vi "Begin.vi"() -> (0 "error out":errorcluster)   [LabVIEW 2012]
doc: "Called before other user functions, this VI is expected to open initial I/O refnums, load in file data, and do all program initialization. Notice that the <B>error out</B> terminal is simply used for data flow. Wiring it to other structures or subVIs ensures that this VI runs first."
uses:
  <vilib>/Rock Robotics/WPI/DriverStation/WPI_DriverStationRobotMode2.ctl
  <vilib>/Rock Robotics/WPI/Joystick/WPI_JoystickDeviceEnum.ctl
  <vilib>/Rock Robotics/WPI/Solenoid/WPI_SolenoidChannel.ctl
  <vilib>/Rock Robotics/SystemInterfaces/DIO/FPGA_DIOChannel.ctl
  <vilib>/Rock Robotics/WPI/Encoder/WPI_EncoderType.ctl
  <vilib>/Rock Robotics/SystemInterfaces/DIO/FPGA_DIOPWMChannel.ctl
  <vilib>/Rock Robotics/SystemInterfaces/DIO/FPGA_DIORelayChannel.ctl
  <vilib>/Rock Robotics/SystemInterfaces/AI/FPGA_AIGyroChannel.ctl
  Robot Global Data.vi
  <vilib>/Rock Robotics/WPI/Solenoid/WPI_SolenoidOpenSingle.vi
  <vilib>/Rock Robotics/WPI/Solenoid/Deprecated/WPI_SolenoidSetBool.vi
  <vilib>/Rock Robotics/WPI/Counter/WPI_CounterDigitalInputToDigitalSource.vi
  <vilib>/Rock Robotics/WPI/MotorControl/WPI_MotorControlOpen Jaguar.vi
  <vilib>/Rock Robotics/WPI/RobotDrive/WPI_RobotDriveOpen4MotorWithTalon.vi
  <vilib>/Rock Robotics/WPI/Compressor/WPI_CompressorGetSetRefNum.vi
  <vilib>/Rock Robotics/WPI/MotorControl/WPI_MotorControlOpen Talon.vi
  <vilib>/Rock Robotics/WPI/MotorControl/WPI_MotorControlOpen Victor.vi
  <vilib>/Rock Robotics/WPI/RobotDrive/WPI_RobotDriveOpen4MotorWithExistingMotors.vi
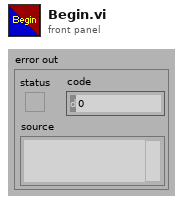
[diagram p1: front panel]
types:
  T1 = typedef "FPGA_DIOPWMChannel.ctl" = enum8{"PWM 1", "PWM 2", "PWM 3", "PWM 4", "PWM 5", "PWM 6", "PWM 7", "PWM 8", "PWM 9", "PWM 10", "Invalid"}
  T2 = typedef "FPGA_DIOChannel.ctl" = enum8{"DIO 1", "DIO 2", "DIO 3", "DIO 4", "DIO 5", "DIO 6", "DIO 7", "DIO 8", "DIO 9", "DIO 10", "DIO 11", "DIO 12", "DIO 13", "DIO 14", "Invalid"}
  T3 = typedef "WPI_SolenoidChannel.ctl" = enum8{"Solenoid 1", "Solenoid 2", "Solenoid 3", "Solenoid 4", "Solenoid 5", "Solenoid 6", "Solenoid 7", "Solenoid 8", "Invalid"}
  T4 = typedef "FPGA_AIGyroChannel.ctl" = enum8{"AI 1", "AI 2", "Invalid"}
  T5 = typedef "WPI_EncoderType.ctl" = enum16{"1x", "2x", "4x"}
  T6 = typedef "FPGA_DIORelayChannel.ctl" = enum8{"Relay 1", "Relay 2", "Relay 3", "Relay 4", "Relay 5", "Relay 6", "Relay 7", "Relay 8", "Invalid"}
  T7 = typedef "WPI_JoystickDeviceEnum.ctl" = enum16{"USB 1", "USB 2", "USB 3", "USB 4", "Kinect 1", "Kinect 2"}
  T8 = typedef "WPI_DriverStationRobotMode2.ctl" = enum16{"Autonomous Disabled", "Autonomous Enabled", "Teleop Disabled", "Teleop Enabled", "Timeout", "Finish", "Test Disabled", "Test Enabled"}
  T9 = typedef "WPI_RobotDriveDevRef.ctl" = cluster{"DevStatus":errorcluster, "Motors[]":T10[], "Square Inputs":bool, "Max Output":dbl, "Isochronous":bool}
  T10 = typedef "WPI_MotorControlDeviceRef.ctl" = cluster{"DeviceStatus":errorcluster, "Type":enum16{"PWM", "CAN"}, "PWM":cluster{"Digital Module":T11, "PWM Channel":T1, "DeadBand":T12}, "CAN":cluster{"Device Number":u8, "Control Mode":T13, "Semaphore":T14, "Max Vout":dbl}, "Invert":bool, "TransformRef":T15, "InvTransformRef":T15}
  T11 = typedef "FPGA_TypedefDigitalModule.ctl" = enum16{"Digital Module 1", "Digital Module 2"}
  T12 = typedef "WPI_PWMDeadband.ctl" = cluster{"Name":string, "maxPositivePwm":i32, "minPositivePwm":i32, "centerPwm":i32, "maxNegativePwm":i32, "minNegativePwm":i32, "angularRange":u16}
  T13 = typedef "WPI_CANJaguar_ControlMode.ctl" = enum8{"Percent VBus", "Current", "Speed", "Position", "Voltage"}
  T14 = typedef "Semaphore RefNum" = refnum<k1>
  T15 = typedef "WPI_PWMTransform_ConPane.ctl" = refnum<vi>
  T16 = typedef "WPI_CompressorDevRef.ctl" = cluster{"DevStatus":errorcluster, "DigitalInputDevRef":T17, "RelayDevRef":T18}
  T17 = typedef "WPI_DigitalInputDevRef.ctl" = cluster{"DevStatus":errorcluster, "DIO Channel":T2, "Digital Module":T11}
  T18 = typedef "WPI_RelayDevRef.ctl" = cluster{"DevStatus":errorcluster, "Relay Channel":T6, "Digital Module":T11, "Relay Direction":T19}
  T19 = typedef "WPI_RelayDirection.ctl" = enum16{"Both directions", "Forward only", "Reverse only"}
  T20 = typedef "WPI_JoystickDevRef.ctl" = cluster{"Device":T7}
  T21 = typedef "WPI_ServoDeviceRef.ctl" = cluster{"DeviceStatus":errorcluster, "Digital Module":T11, "PWM Channel":T1, "DeadBand":T12}
  T22 = typedef "WPI_SolenoidDevRef.ctl" = cluster{"DevStatus":errorcluster, "Solenoid Module":T23, "Forward Solenoid Channel":T3, "Reverse Solenoid Channel":T3}
  T23 = typedef "FPGA_TypedefSolenoidModule.ctl" = enum16{"Solenoid Module 1", "Solenoid Module 2"}
  T24 = typedef "FPGA_CounterEncoderSourceConvertionLVSourceType.ctl" = cluster{"DevStatus":errorcluster, "AnalogTriggerMode?":bool, "DigitalMode":cluster{"Digital Module":T11, "DIO Channel":T25}, "AnalogTriggerMode":cluster{"AnalogTriggerIndex":T26, "OutputType":T27}}
  T25 = typedef "FPGA_DIODigitalSourceChannel.ctl" = enum8{"DIO 1", "DIO 2", "DIO 3", "DIO 4", "DIO 5", "DIO 6", "DIO 7", "DIO 8", "DIO 9", "DIO 10", "DIO 11", "DIO 12", "DIO 13", "DIO 14", "Disabled"}
  T26 = typedef "FPGA_AnalogTriggerIndex.ctl" = enum8{"Trig 0", "Trig 1", "Trig 2", "Trig 3", "Trig 4", "Trig 5", "Trig 6", "Trig 7", "Invalid"}
  T27 = typedef "FPGA_AnalogTriggerOutType.ctl" = enum16{"InWindow", "TriggerState", "Rising", "Falling"}
  T28 = typedef "WPI_GyroDevRef.ctl" = cluster{"DevStatus":errorcluster, "Analog Module":T29, "Analog Channel":T30, "Offset":dbl, "Gain (VoltsPerDegree/Second)":dbl}
  T29 = typedef "FPGA_TypedefAnalogModule.ctl" = enum16{"Analog Module 1", "Analog Module 2"}
  T30 = typedef "FPGA_AIChannel.ctl" = enum8{"AI 1", "AI 2", "AI 3", "AI 4", "AI 5", "AI 6", "AI 7", "AI 8", "Invalid"}
  T31 = typedef "WPI_EncoderDevRef.ctl" = cluster{"DevStatus":errorcluster, "EncoderIndex":T32, "CounterIndex":T33, "DistancePerCount":dbl, "Decoding Type":T5}
  T32 = typedef "FPGA_EncoderIdx.ctl" = enum8{"Enc 0", "Enc 1", "Enc 2", "Enc 3", "Invalid"}
  T33 = typedef "FPGA_CounterCtrSystemIndex.ctl" = enum8{"Ctr 0", "Ctr 1", "Ctr 2", "Ctr 3", "Ctr 4", "Ctr 5", "Ctr 6", "Ctr 7", "Invalid"}
  T34 = cluster{"Target Voltage":dbl, "Target Speed":dbl, "Angle Up?":bool}
  T35 = cluster{"Target Voltage":dbl, "Target Speed":i32, "Angle Up?":bool}
  T36 = cluster{"Target Voltage":i32, "Target Speed":i32, "Angle Up?":bool}
  T37 = cluster{"Target Voltage":dbl, "Target Speed":dbl, "Angle Up?":bool}[]
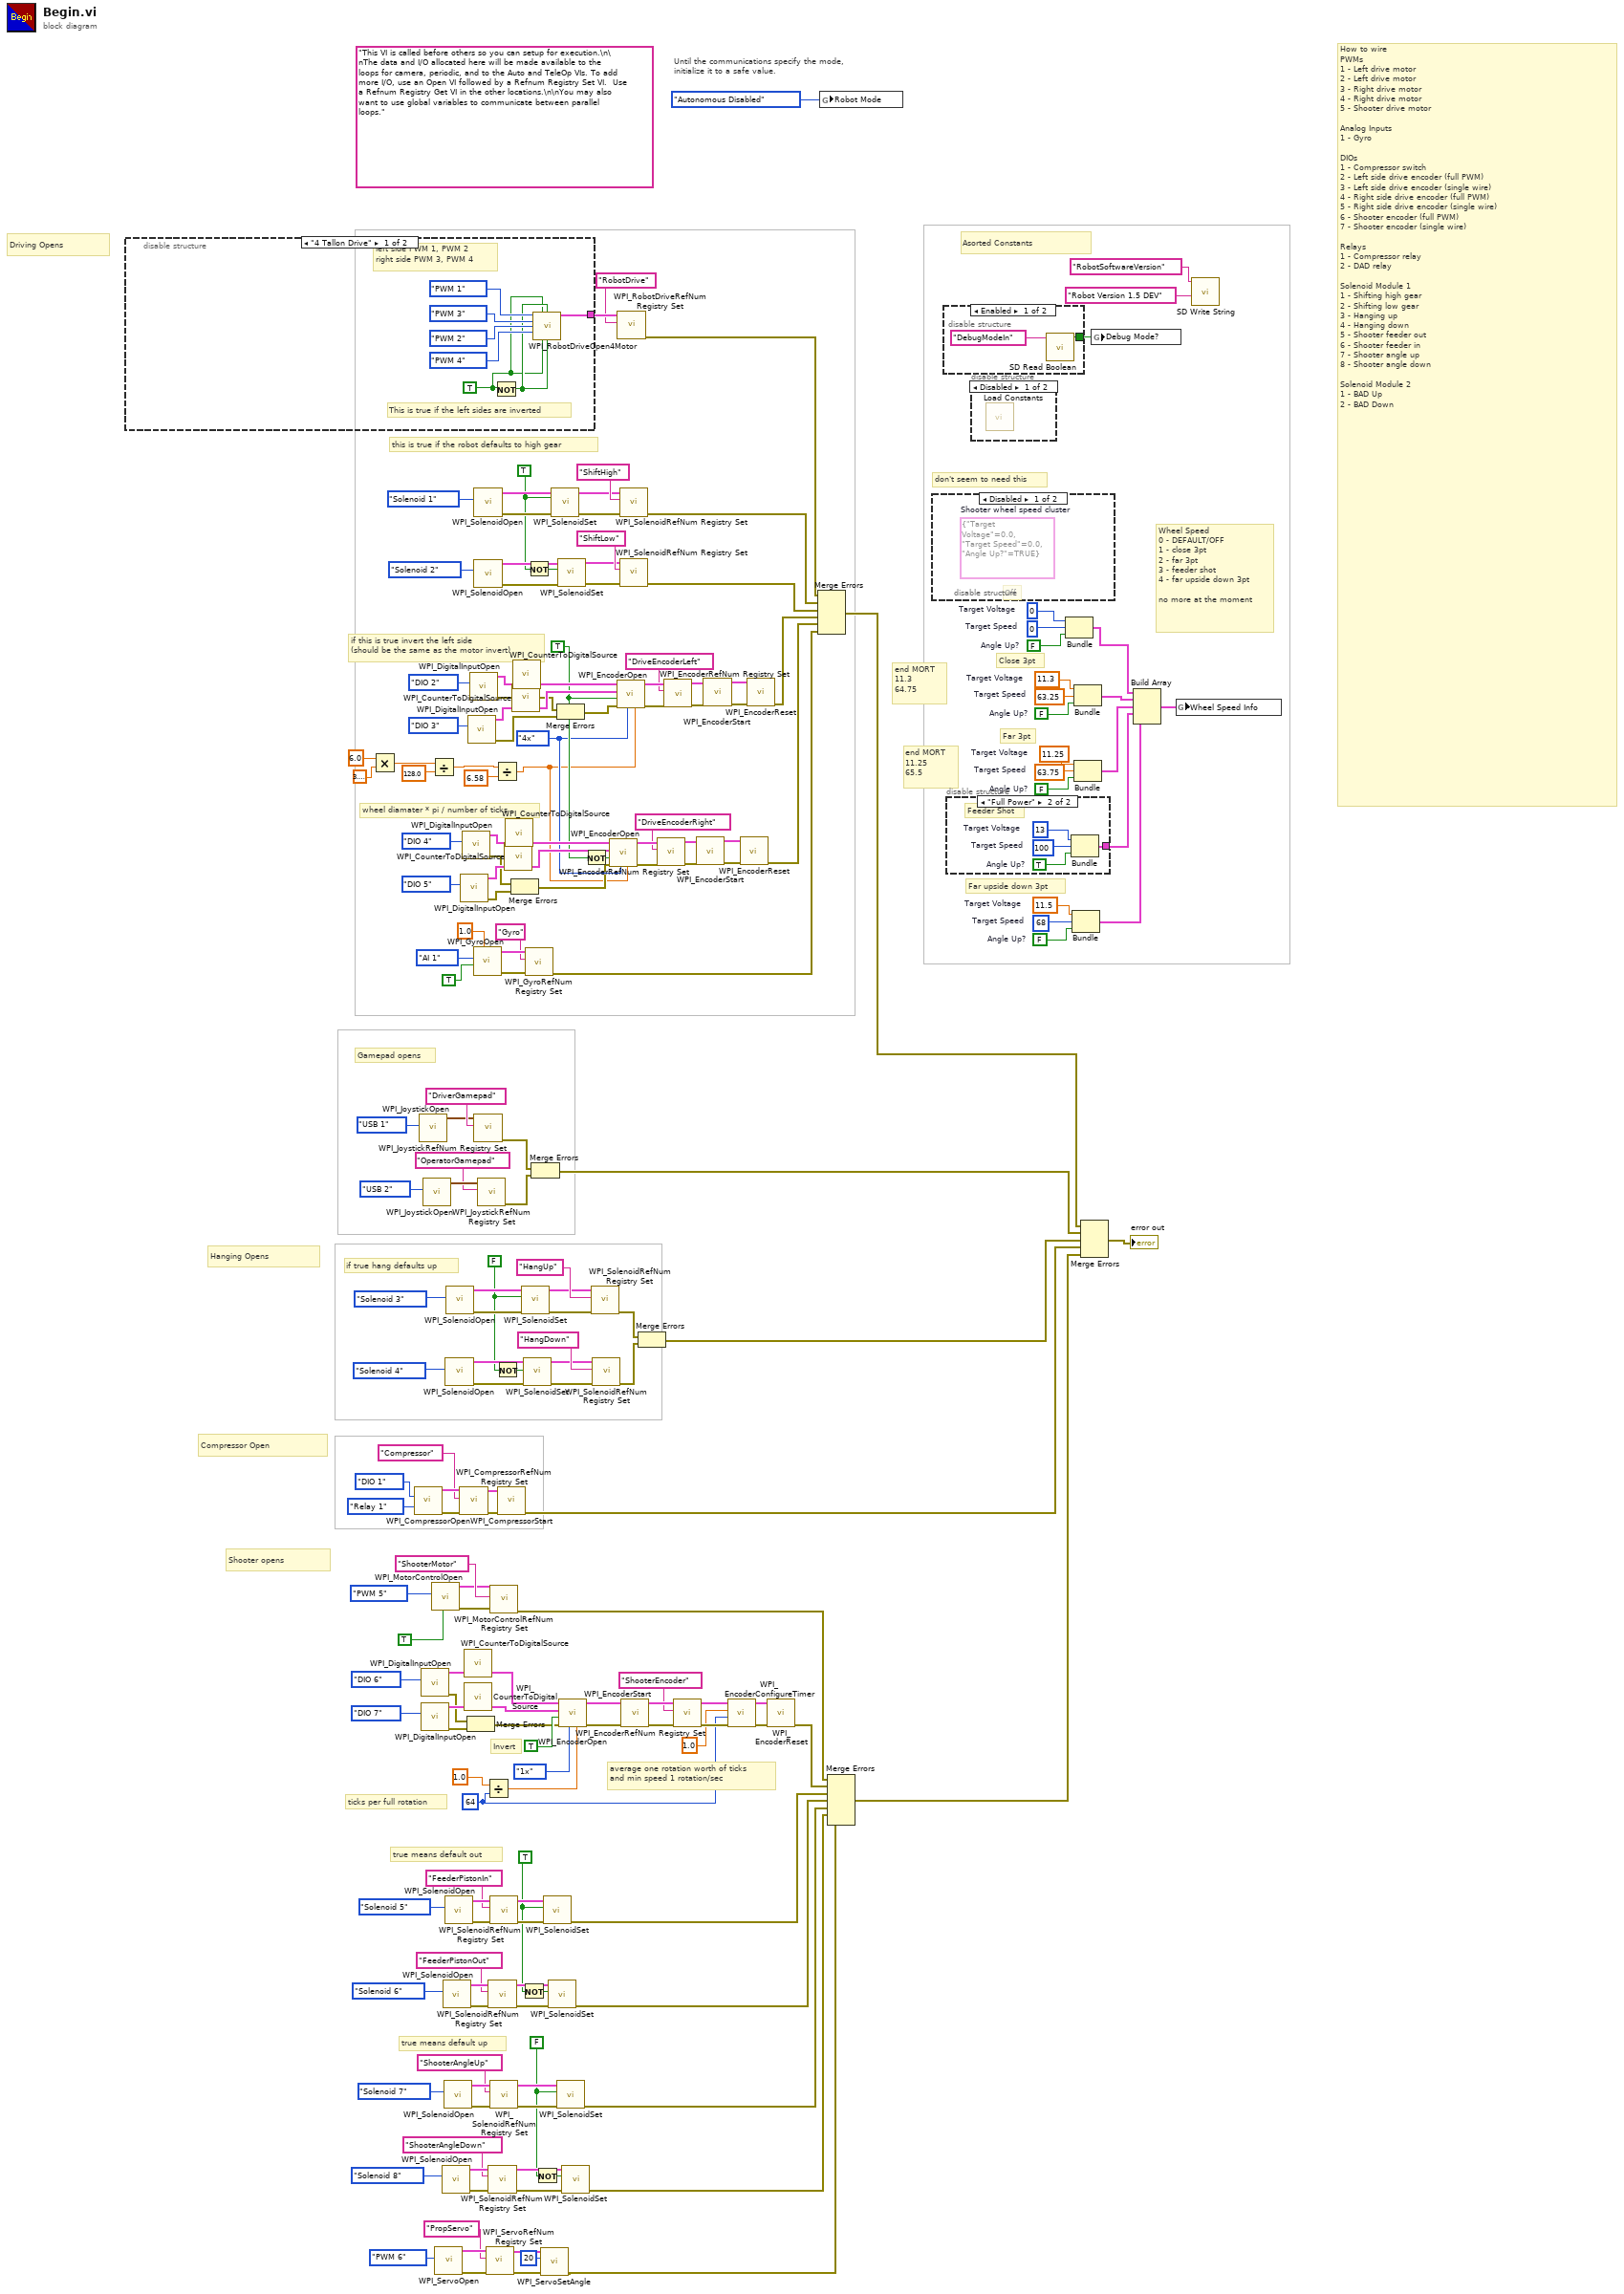
[diagram p0: block diagram]
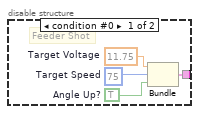
[diagram p3: hidden frame]
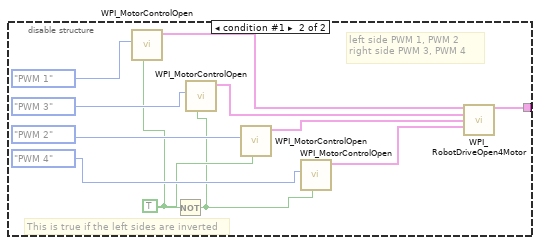
[diagram p4: hidden frame]
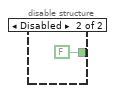
[diagram p5: hidden frame]
diagram:
  w1 = FALSE
  w16 = FALSE  # Angle Up?
  w15 = 63.75  # Target Speed
  w14 = 11.25  # Target Voltage
  w20 = FALSE  # Angle Up?
  w19 = 68  # Target Speed
  w18 = 11.5  # Target Voltage
  w24 = FALSE  # Angle Up?
  w23 = 0  # Target Speed
  w22 = 0  # Target Voltage
  w26 = u8 64 ("Number Samples to Average")
  w33 = FALSE  # Angle Up?
  w34 = 63.25  # Target Speed
  w35 = 11.3  # Target Voltage
  w99 = TRUE
  w66 = FALSE
  w68 = WPI_EncoderType."4x" ("Decoding Type")
  w69 = TRUE ("Invert Direction (False)")
  w85 = TRUE
  (unwired) "This VI is called before others so you can setup for execution.\n\nThe data and I/O allocated here will be made available to the loops for camera, periodic, and to the Auto and TeleOp VIs. To add more I/O, use an Open VI followed by a Refnum Registry Set VI.  Use a Refnum Registry Get VI in the other locations.\n\nYou may also want to use global variables to communicate between parallel loops."
  # "end MORT\n11.3\n64.75"
  # "end MORT\n11.25\n65.5"
  # "don't seem to need this"
  # "Far 3pt"
  # "Far upside down 3pt"
  # "average one rotation worth of ticks\nand min speed 1 rotation/sec"
  # "Close 3pt"
  # "How to wire\nPWMs\n1 - Left drive motor\n2 - Left drive motor\n3 - Right drive motor\n4 - Right drive motor\n5 - Shooter drive motor\n\nAnalog Inputs\n1 - Gyro\n\nDIOs\n1 - Compressor switch\n2 - Left side drive encoder (full PWM)\n3 - Left side drive encoder (single wire)\n4 - Right side drive encoder (full PWM)\n5 - Right side drive encoder (single wire)\n6 - Shooter encoder (full PWM)\n7 - Shooter encoder (single wire)\n\nRelays\n1 - Compressor relay\n2 - DAD relay\n\nSolenoid Module 1\n1 - Shifting high gear\n2 - Shifting low gear\n3 - Hanging up\n4 - Hanging down\n5 - Shooter feeder out\n6 - Shooter feeder in\n7 - Shooter angle up\n8 - Shooter angle down\n\nSolenoid Module 2\n1 - BAD Up\n2 - BAD Down"
  # "Asorted Constants"
  # "true means default up"
  # "true means default out"
  # "if true hang defaults up"
  # "Gamepad opens"
  # "wheel diamater * pi / number of ticks"
  # "if this is true invert the left side\n(should be the same as the motor invert)"
  # "this is true if the robot defaults to high gear"
  # "Compressor Open"
  # "Wheel Speed\n0 - DEFAULT/OFF\n1 - close 3pt\n2 - far 3pt\n3 - feeder shot\n4 - far upside down 3pt\n\nno more at the moment"
  # "Hanging Opens"
  # "Driving Opens"
  # "Shooter opens"
  # "Invert"
  # "ticks per full rotation"
  # "Until the communications specify the mode,\ninitialize it to a safe value."
  n1 = disable-structure shown="\"4 Tallon Drive\"" {
    disable-tunnel: [w203 w218] -> w196
    frame condition #0 (active) {
      w201 = TRUE ("Rear Left Motor Inverted")
      # "left side PWM 1, PWM 2\nright side PWM 3, PWM 4"
      # "This is true if the left sides are inverted"
      n2 = Not(x=w201) -> (.not. x?=w202:bool)
      n3 = call-poly <vilib>:"WPI_RobotDriveOpen4Motor.vi"("Rear Left Motor"=FPGA_DIOPWMChannel."PWM 1", "Rear Left Motor Inverted"=w201, "Rear Right Motor Inverted"=w202, "Rear Right Motor"=FPGA_DIOPWMChannel."PWM 3", "Front Left Motor"=FPGA_DIOPWMChannel."PWM 2", "Front Right Motor"=FPGA_DIOPWMChannel."PWM 4" ("Front Left Motor"), "Front Left Motor Inverted"=w201, "Front Right Motor Inverted"=w202) -> ("RobotDriveDevRef"=w203:T9)  [unwired: 6 in, 1 out]
    }
    frame condition #1 {
      w213 = TRUE ("Rear Left Motor Inverted")
      # "left side PWM 1, PWM 2\nright side PWM 3, PWM 4"
      # "This is true if the left sides are inverted"
      n4 = call-poly <vilib>:"WPI_MotorControlOpen.vi"("Invert"=w213, "PWM Channel"=FPGA_DIOPWMChannel."PWM 1" ("Rear Left Motor")) -> ("MotorControlDeviceRef"=w211:T10)  [unwired: 8 in, 1 out]
      n5 = Not(x=w213) -> (.not. x?=w212:bool)
      n6 = call-poly <vilib>:"WPI_MotorControlOpen.vi"("Invert"=w212, "PWM Channel"=FPGA_DIOPWMChannel."PWM 3" ("Rear Right Motor")) -> ("MotorControlDeviceRef"=w210:T10)  [unwired: 8 in, 1 out]
      n7 = call-poly <vilib>:"WPI_MotorControlOpen.vi"("Invert"=w213, "PWM Channel"=FPGA_DIOPWMChannel."PWM 2" ("Front Left Motor")) -> ("MotorControlDeviceRef"=w209:T10)  [unwired: 8 in, 1 out]
      n8 = call-poly <vilib>:"WPI_MotorControlOpen.vi"("Invert"=w212, "PWM Channel"=FPGA_DIOPWMChannel."PWM 4" ("Front Left Motor")) -> ("MotorControlDeviceRef"=w208:T10)  [unwired: 8 in, 1 out]
      n9 = call-poly <vilib>:"WPI_RobotDriveOpen4Motor.vi"("Rear Left Motor Dev Ref"=w211, "Rear Right Motor Dev Ref"=w210, "Front Left Motor Dev Ref"=w209, "Front Right Motor Dev Ref"=w208) -> ("RobotDriveDevRef"=w218:T9)  [unwired: 10 in, 1 out]
    }
  }
  n10 = Multiply(x=6.0, y=3.141592653589793) -> (x*y=w140:dbl)
  n11 = call <vilib>:"WPI_CompressorOpen.vi"("Pressure Switch DIO Channel"=FPGA_DIOChannel."DIO 1", "Relay Channel"=FPGA_DIORelayChannel."Relay 1") -> ("CompressorDevRef"=w153:T16, "error out"=w151:errorcluster)  [unwired: 12 in]
  n12 = call <vilib>:"WPI_JoystickOpen.vi"("JoystickDevice"=WPI_JoystickDeviceEnum."USB 1") -> ("JoystickDevRef"=w198:T20)  [unwired: 10 in]
  n13 = call <vilib>:"WPI_DigitalInputOpen.vi"("DIO Channel"=FPGA_DIOChannel."DIO 6") -> ("error out"=w169:errorcluster, "DigitalInputDevRef"=w182:T17)  [unwired: 9 in]
  n14 = call <vilib>:"WPI_DigitalInputOpen.vi"("DIO Channel"=FPGA_DIOChannel."DIO 7") -> ("error out"=w168:errorcluster, "DigitalInputDevRef"=w178:T17)  [unwired: 9 in]
  n15 = call <vilib>:"WPI_JoystickOpen.vi"("JoystickDevice"=WPI_JoystickDeviceEnum."USB 2") -> ("JoystickDevRef"=w155:T20)  [unwired: 10 in]
  n16 = Divide(x=w140, y=128.0 ("x")) -> (x/y=w12:dbl)
  n17 = call-poly <vilib>:"WPI_MotorControlOpen.vi"("Invert"=TRUE, "PWM Channel"=FPGA_DIOPWMChannel."PWM 5") -> ("error out"=w162:errorcluster, "MotorControlDeviceRef"=w163:T10)  [unwired: 8 in]
  n18 = call <vilib>:"WPI_ServoOpen.vi"("PWM Channel"=FPGA_DIOPWMChannel."PWM 6") -> ("error out"=w8:errorcluster, "ServoDeviceRef"=w10:T21)  [unwired: 9 in]
  n19 = call-poly <vilib>:"WPI_SolenoidOpen.vi"("Solenoid Channel"=WPI_SolenoidChannel."Solenoid 8") -> ("error out"=w96:errorcluster, "SolenoidDevRef"=w95:T22)  [unwired: 9 in]
  n20 = call-poly <vilib>:"WPI_SolenoidOpen.vi"("Solenoid Channel"=WPI_SolenoidChannel."Solenoid 6") -> ("error out"=w109:errorcluster, "SolenoidDevRef"=w108:T22)  [unwired: 9 in]
  n21 = call-poly <vilib>:"WPI_SolenoidOpen.vi"("Solenoid Channel"=WPI_SolenoidChannel."Solenoid 7") -> ("error out"=w91:errorcluster, "SolenoidDevRef"=w92:T22)  [unwired: 9 in]
  n22 = call-poly <vilib>:"WPI_SolenoidOpen.vi"("Solenoid Channel"=WPI_SolenoidChannel."Solenoid 5") -> ("error out"=w104:errorcluster, "SolenoidDevRef"=w105:T22)  [unwired: 9 in]
  n23 = call-poly <vilib>:"WPI_SolenoidOpen.vi"("Solenoid Channel"=WPI_SolenoidChannel."Solenoid 4") -> ("error out"=w119:errorcluster, "SolenoidDevRef"=w120:T22)  [unwired: 9 in]
  n24 = call-poly <vilib>:"WPI_SolenoidOpen.vi"("Solenoid Channel"=WPI_SolenoidChannel."Solenoid 3") -> ("error out"=w122:errorcluster, "SolenoidDevRef"=w121:T22)  [unwired: 9 in]
  n25 = call <vilib>:"WPI_CompressorRefNum Registry Set.vi"("error in (no error)"=w151, "refnum name"="Compressor", "CompressorDevRef"=w153) -> ("error out"=w113:errorcluster, "CompressorDevRef"=w114:T16)  [unwired: 7 in]
  n26 = call <vilib>:"WPI_DigitalInputOpen.vi"("DIO Channel"=FPGA_DIOChannel."DIO 5") -> ("error out"=w59:errorcluster, "DigitalInputDevRef"=w77:T17)  [unwired: 9 in]
  n27 = call <vilib>:"WPI_DigitalInputOpen.vi"("DIO Channel"=FPGA_DIOChannel."DIO 4") -> ("error out"=w58:errorcluster, "DigitalInputDevRef"=w76:T17)  [unwired: 9 in]
  n28 = call-poly <vilib>:"WPI_CounterToDigitalSource.vi"("DigitalInputDevRef"=w182) -> ("Digital Source"=w181:T24)  [unwired: 6 in]
  n29 = call-poly <vilib>:"WPI_CounterToDigitalSource.vi"("DigitalInputDevRef"=w178) -> ("Digital Source"=w175:T24)  [unwired: 6 in]
  n30 = Merge Errors(w169, w168) -> (w170:errorcluster)
  n31 = call <vilib>:"WPI_DigitalInputOpen.vi"("DIO Channel"=FPGA_DIOChannel."DIO 3") -> ("error out"=w54:errorcluster, "DigitalInputDevRef"=w143:T17)  [unwired: 9 in]
  n32 = call <vilib>:"WPI_DigitalInputOpen.vi"("DIO Channel"=FPGA_DIOChannel."DIO 2") -> ("error out"=w55:errorcluster, "DigitalInputDevRef"=w144:T17)  [unwired: 9 in]
  n33 = call <vilib>:"WPI_GyroOpen.vi"("Calibration Time (s)"=1.0, "Calibrate On Open"=TRUE, "Analog Channel"=FPGA_AIGyroChannel."AI 1") -> ("error out"=w132:errorcluster, "GyroDevRef"=w131:T28)  [unwired: 6 in, 1 out]
  n34 = call-poly <vilib>:"WPI_SolenoidOpen.vi"("Solenoid Channel"=WPI_SolenoidChannel."Solenoid 1") -> ("error out"=w187:errorcluster, "SolenoidDevRef"=w190:T22)  [unwired: 9 in]
  n35 = call-poly <vilib>:"WPI_SolenoidOpen.vi"("Solenoid Channel"=WPI_SolenoidChannel."Solenoid 2") -> ("error out"=w184:errorcluster, "SolenoidDevRef"=w186:T22)  [unwired: 9 in]
  n36 = call <vilib>:"WPI_JoystickRefNum Registry Set.vi"("refnum name"="DriverGamepad", "JoystickDevRef"=w198) -> ("error out"=w51:errorcluster)  [unwired: 8 in, 1 out]
  n37 = call <vilib>:"WPI_JoystickRefNum Registry Set.vi"("refnum name"="OperatorGamepad", "JoystickDevRef"=w155) -> ("error out"=w50:errorcluster)  [unwired: 8 in, 1 out]
  n38 = Divide(x=1.0, y=w26) -> (x/y=w27:dbl)
  n39 = call <vilib>:"WPI_ServoRefNum Registry Set.vi"("error in (no error)"=w8, "refnum name"="PropServo", "ServoDeviceRef"=w10) -> ("error out"=w5:errorcluster, "ServoDeviceRef"=w4:T21)  [unwired: 7 in]
  n40 = call <vilib>:"WPI_SolenoidRefNum Registry Set.vi"("error in (no error)"=w109, "refnum name"="FeederPistonOut", "SolenoidDevRef"=w108) -> ("error out"=w111:errorcluster, "SolenoidDevRef"=w110:T22)  [unwired: 7 in]
  n41 = call <vilib>:"WPI_SolenoidRefNum Registry Set.vi"("error in (no error)"=w96, "refnum name"="ShooterAngleDown", "SolenoidDevRef"=w95) -> ("error out"=w98:errorcluster, "SolenoidDevRef"=w97:T22)  [unwired: 7 in]
  n42 = call <vilib>:"WPI_MotorControlRefNum Registry Set.vi"("error in (no error)"=w162, "refnum name"="ShooterMotor", "MotorControlDevRef"=w163) -> ("error out"=w47:errorcluster)  [unwired: 7 in, 1 out]
  n43 = call <vilib>:"WPI_SolenoidRefNum Registry Set.vi"("error in (no error)"=w104, "refnum name"="FeederPistonIn", "SolenoidDevRef"=w105) -> ("error out"=w102:errorcluster, "SolenoidDevRef"=w103:T22)  [unwired: 7 in]
  n44 = call <vilib>:"WPI_SolenoidRefNum Registry Set.vi"("error in (no error)"=w91, "refnum name"="ShooterAngleUp", "SolenoidDevRef"=w92) -> ("error out"=w89:errorcluster, "SolenoidDevRef"=w90:T22)  [unwired: 7 in]
  n45 = Divide(x=w12, y=6.58 ("x")) -> (x/y=w13:dbl)
  n46 = Not(x=w66) -> (.not. x?=w67:bool)
  n47 = call <vilib>:"WPI_CompressorStart.vi"("error in (no error)"=w113, "CompressorDevRef"=w114) -> ("error out"=w38:errorcluster)  [unwired: 8 in, 1 out]
  n48 = call-poly <vilib>:"WPI_CounterToDigitalSource.vi"("DigitalInputDevRef"=w77) -> ("Digital Source"=w74:T24)  [unwired: 6 in]
  n49 = call-poly <vilib>:"WPI_CounterToDigitalSource.vi"("DigitalInputDevRef"=w76) -> ("Digital Source"=w72:T24)  [unwired: 6 in]
  n50 = Merge Errors(w58, w59) -> (w57:errorcluster)
  n51 = call-poly <vilib>:"WPI_CounterToDigitalSource.vi"("DigitalInputDevRef"=w143) -> ("Digital Source"=w146:T24)  [unwired: 6 in]
  n52 = call-poly <vilib>:"WPI_CounterToDigitalSource.vi"("DigitalInputDevRef"=w144) -> ("Digital Source"=w148:T24)  [unwired: 6 in]
  n53 = Not(x=w99) -> (.not. x?=w112:bool)
  n54 = call-poly <vilib>:"WPI_SolenoidSet.vi"("error in (no error)"=w122, "Value"=w66, "SolenoidDevRef"=w121) -> ("error out"=w115:errorcluster, "SolenoidDevRef"=w118:T22)  [unwired: 7 in]
  n55 = call-poly <vilib>:"WPI_SolenoidSet.vi"("error in (no error)"=w119, "Value"=w67, "SolenoidDevRef"=w120) -> ("error out"=w116:errorcluster, "SolenoidDevRef"=w117:T22)  [unwired: 7 in]
  n56 = Not(x=w85) -> (.not. x?=w86:bool)
  n57 = call <vilib>:"WPI_GyroRefNum Registry Set.vi"("error in (no error)"=w132, "refnum name"="Gyro", "GyroDevRef"=w131) -> ("error out"=w52:errorcluster)  [unwired: 7 in, 1 out]
  n58 = Merge Errors(w51, w50) -> (w40:errorcluster)
  n59 = Not(x=w1) -> (.not. x?=w2:bool)
  n60 = call <vilib>:"WPI_ServoSetAngle.vi"("error in (no error)"=w5, "Angle"=20, "ServoDeviceRef"=w4) -> ("error out"=w6:errorcluster)  [unwired: 7 in, 1 out]
  n61 = call-poly <vilib>:"WPI_SolenoidSet.vi"("error in (no error)"=w102, "Value"=w99, "SolenoidDevRef"=w103) -> ("error out"=w45:errorcluster)  [unwired: 7 in, 1 out]
  n62 = call-poly <vilib>:"WPI_SolenoidSet.vi"("error in (no error)"=w111, "Value"=w112, "SolenoidDevRef"=w110) -> ("error out"=w44:errorcluster)  [unwired: 7 in, 1 out]
  n63 = call-poly <vilib>:"WPI_SolenoidSet.vi"("error in (no error)"=w187, "Value"=w85, "SolenoidDevRef"=w190) -> ("error out"=w188:errorcluster, "SolenoidDevRef"=w189:T22)  [unwired: 7 in]
  n64 = Merge Errors(w55, w54) -> (w56:errorcluster)
  n65 = call-poly <vilib>:"WPI_SolenoidSet.vi"("error in (no error)"=w89, "Value"=w1, "SolenoidDevRef"=w90) -> ("error out"=w43:errorcluster)  [unwired: 7 in, 1 out]
  n66 = call-poly <vilib>:"WPI_SolenoidSet.vi"("error in (no error)"=w184, "Value"=w86, "SolenoidDevRef"=w186) -> ("error out"=w183:errorcluster, "SolenoidDevRef"=w185:T22)  [unwired: 7 in]
  n67 = call <vilib>:"WPI_EncoderOpen.vi"("DistancePerCount"=w27, "Decoding Type"=WPI_EncoderType."1x", "error in (no error)"=w170, "Invert Direction (False)"=TRUE, "BSource"=w175, "ASource"=w181) -> ("error out"=w171:errorcluster, "EncoderDevRef"=w172:T31)  [unwired: 4 in]
  n68 = call-poly <vilib>:"WPI_SolenoidSet.vi"("error in (no error)"=w98, "Value"=w2, "SolenoidDevRef"=w97) -> ("error out"=w42:errorcluster)  [unwired: 7 in, 1 out]
  n69 = Not(x=w69) -> (.not. x?=w70:bool)
  n70 = call <vilib>:"WPI_SolenoidRefNum Registry Set.vi"("error in (no error)"=w115, "refnum name"="HangUp", "SolenoidDevRef"=w118) -> ("error out"=w49:errorcluster)  [unwired: 7 in, 1 out]
  n71 = call <vilib>:"WPI_SolenoidRefNum Registry Set.vi"("error in (no error)"=w116, "refnum name"="HangDown", "SolenoidDevRef"=w117) -> ("error out"=w48:errorcluster)  [unwired: 7 in, 1 out]
  n72 = call <vilib>:"WPI_EncoderOpen.vi"("DistancePerCount"=w13, "Decoding Type"=w68, "error in (no error)"=w57, "Invert Direction (False)"=w70, "BSource"=w74, "ASource"=w72) -> ("error out"=w78:errorcluster, "EncoderDevRef"=w79:T31)  [unwired: 4 in]
  n73 = call <vilib>:"WPI_EncoderOpen.vi"("DistancePerCount"=w13, "Decoding Type"=w68, "error in (no error)"=w56, "Invert Direction (False)"=w69, "BSource"=w146, "ASource"=w148) -> ("error out"=w139:errorcluster, "EncoderDevRef"=w138:T31)  [unwired: 4 in]
  n74 = call <vilib>:"WPI_RobotDriveRefNum Registry Set.vi"("refnum name"="RobotDrive", "RobotDriveDevRef"=w196) -> ("error out"=w63:errorcluster)  [unwired: 8 in, 1 out]
  n75 = call <vilib>:"WPI_SolenoidRefNum Registry Set.vi"("error in (no error)"=w188, "refnum name"="ShiftHigh", "SolenoidDevRef"=w189) -> ("error out"=w62:errorcluster)  [unwired: 7 in, 1 out]
  n76 = call <vilib>:"WPI_SolenoidRefNum Registry Set.vi"("error in (no error)"=w183, "refnum name"="ShiftLow", "SolenoidDevRef"=w185) -> ("error out"=w61:errorcluster)  [unwired: 7 in, 1 out]
  n77 = call <vilib>:"WPI_EncoderStart.vi"("error in (no error)"=w171, "EncoderDevRef"=w172) -> ("error out"=w167:errorcluster, "EncoderDevRef"=w173:T31)  [unwired: 8 in]
  n78 = Merge Errors(w49, w48) -> (w39:errorcluster)
  n79 = call <vilib>:"WPI_EncoderRefNum Registry Set.vi"("error in (no error)"=w78, "refnum name"="DriveEncoderRight", "EncoderDevRef"=w79) -> ("error out"=w80:errorcluster, "EncoderDevRef"=w81:T31)  [unwired: 7 in]
  n80 = call <vilib>:"WPI_EncoderRefNum Registry Set.vi"("error in (no error)"=w139, "refnum name"="DriveEncoderLeft", "EncoderDevRef"=w138) -> ("error out"=w137:errorcluster, "EncoderDevRef"=w136:T31)  [unwired: 7 in]
  n81 = call <vilib>:"WPI_EncoderRefNum Registry Set.vi"("error in (no error)"=w167, "refnum name"="ShooterEncoder", "EncoderDevRef"=w173) -> ("error out"=w158:errorcluster, "EncoderDevRef"=w159:T31)  [unwired: 7 in]
  n82 = call <vilib>:"WPI_EncoderStart.vi"("error in (no error)"=w80, "EncoderDevRef"=w81) -> ("error out"=w82:errorcluster, "EncoderDevRef"=w83:T31)  [unwired: 8 in]
  n83 = call <vilib>:"WPI_EncoderStart.vi"("error in (no error)"=w137, "EncoderDevRef"=w136) -> ("error out"=w135:errorcluster, "EncoderDevRef"=w134:T31)  [unwired: 8 in]
  n84 = call <vilib>:"WPI_EncoderConfigureTimer.vi"("error in (no error)"=w158, "Number Samples to Average"=w26, "Minimum Rate"=1.0, "EncoderDevRef"=w159) -> ("error out"=w161:errorcluster, "EncoderDevRef"=w160:T31)  [unwired: 6 in]
  n85 = call <vilib>:"WPI_EncoderReset.vi"("error in (no error)"=w82, "EncoderDevRef"=w83) -> ("error out"=w53:errorcluster)  [unwired: 8 in, 1 out]
  n86 = call <vilib>:"WPI_EncoderReset.vi"("error in (no error)"=w135, "EncoderDevRef"=w134) -> ("error out"=w60:errorcluster)  [unwired: 8 in, 1 out]
  n87 = call <vilib>:"WPI_EncoderReset.vi"("error in (no error)"=w161, "EncoderDevRef"=w160) -> ("error out"=w46:errorcluster)  [unwired: 8 in, 1 out]
  n88 = Merge Errors(w63, w62, w61, w60, w53, w52) -> (w41:errorcluster)
  n89 = global write "Robot Global Data.vi" "Robot Mode"(WPI_DriverStationRobotMode2."Autonomous Disabled" ("Robot Mode")) -> ()
  n90 = Merge Errors(w47, w46, w45, w44, w43, w42, w6) -> (w37:errorcluster)
  n91 = disable-structure shown="Disabled" {
    frame Disabled {
      (unwired) T34 {"Target Voltage"=0.0, "Target Speed"=0.0, "Angle Up?"=TRUE}  # Shooter wheel speed cluster
      # "Off"
    }
    frame Enabled {
    }
  }
  n92 = disable-structure shown="Enabled" {
    disable-tunnel: [w219 FALSE ("Debug Mode?")] -> w28
    frame Enabled {
      n93 = call <vilib>:"SD Read Boolean.vi"("Name"="DebugModeIn") -> ("Boolean"=w219:bool)  [unwired: 8 in, 2 out]
    }
    frame Disabled {
    }
  }
  n94 = disable-structure shown="\"Full Power\"" {
    disable-tunnel: [w222 w226] -> w30
    frame condition #0 {
      w223 = TRUE  # Angle Up?
      w224 = 75  # Target Speed
      w225 = 11.75  # Target Voltage
      # "Feeder Shot"
      n95 = Bundle("Target Voltage"=w225, "Target Speed"=w224, "Angle Up?"=w223) -> (w222:T35)  [unwired: 1 in]
    }
    frame condition #1 (active) {
      w227 = TRUE  # Angle Up?
      w228 = 100  # Target Speed
      w229 = 13  # Target Voltage
      # "Feeder Shot"
      n96 = Bundle("Target Voltage"=w229, "Target Speed"=w228, "Angle Up?"=w227) -> (w226:T36)  [unwired: 1 in]
    }
  }
  n97 = disable-structure shown="Disabled" {
    frame Disabled {
      n98 = call "Load Constants.vi"() -> ()  [unwired: 12 in]
    }
    frame Enabled {
    }
  }
  n99 = Bundle("Target Voltage"=w22, "Target Speed"=w23, "Angle Up?"=w24) -> (w21:T36)  [unwired: 1 in]
  n100 = Bundle("Target Voltage"=w18, "Target Speed"=w19, "Angle Up?"=w20) -> (w17:T35)  [unwired: 1 in]
  n101 = Bundle("Target Voltage"=w35, "Target Speed"=w34, "Angle Up?"=w33) -> (w32:T34)  [unwired: 1 in]
  n102 = Bundle("Target Voltage"=w14, "Target Speed"=w15, "Angle Up?"=w16) -> (w31:T34)  [unwired: 1 in]
  n103 = Merge Errors(w41, w40, w39, w38, w37) -> (→"error out":errorcluster)
  n104 = global write "Robot Global Data.vi" "Debug Mode?"(w28) -> ()
  n105 = Build Array(w21, w32, w31, w30, w17) -> (w29:T37)
  n106 = global write "Robot Global Data.vi" "Wheel Speed Info"(w29) -> ()
  n107 = call <vilib>:"SD Write String.vi"("String"="Robot Version 1.5 DEV", "Name"="RobotSoftwareVersion") -> ()  [unwired: 8 in, 2 out]
